vi "proceso4.vi"() -> ()   [LabVIEW 2020]
panel:
  in  "proceso 4":cluster{"tanque out":u8, "tempertura_final":dbl}
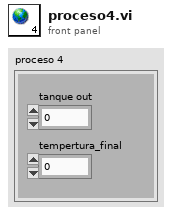
[diagram p1: front panel]
diagram:
